vi "subPortInit.vi"(0 "Control unit ID":i32=1 min=1 max=10) -> (1 "Index":i32, 2 "InitOK":bool)   [LabVIEW 2018, in "DLOwis.lvclass"]
uses:
  DLOwis.lvclass
panel:
  in  "error in (no error)":errorcluster
  out "DLOwis.lvclass":refnum<class "DLOwis.lvclass">
  in  "DLOwis.lvclass":refnum<class "DLOwis.lvclass">
  in  "Timeout":i32 caption="Timeout, ms" min=0
  in  "Network port":u16=1200
  in  "ip4":u8 caption="IP address"
  in  "ip3":u8 caption="IP address"
  in  "ip2":u8 caption="IP address"
  in  "ip1":u8 caption="IP address"
  in  "logging on":bool
  in  "Delay":i32(slide) caption="Fast(0)<--->Slow(50)" min=0 max=50 scale=0.0..50.0
  in  "Baudrate":string(combo)="9600"
  in  "Cancel":bool
  in  "OK":bool
  in  "COM port":i32=-1 caption="COMx" min=-1 max=255
  out "Error":i32
  in  "Interface":bool
  # "Parameters of the interface"
  # "COMx=-1: find\nautomatically"
  # "IP=0.0.0.0: connect\n 1. local ip address \n and port 1200"
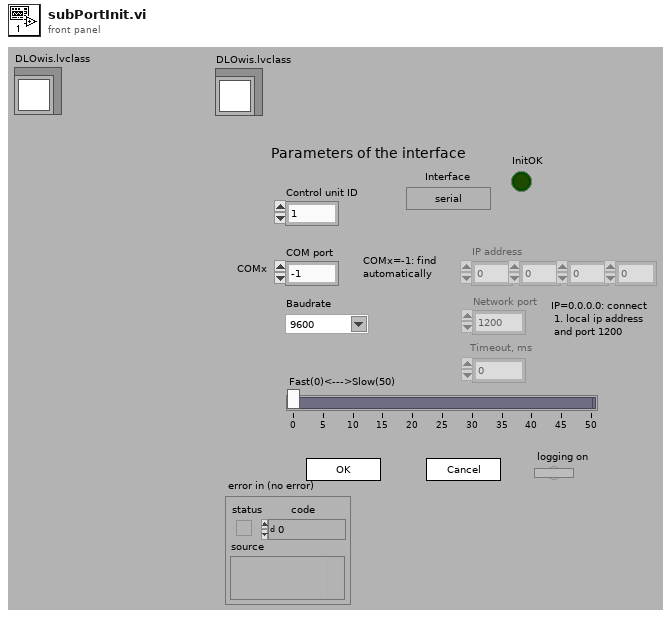
[diagram p1: front panel]
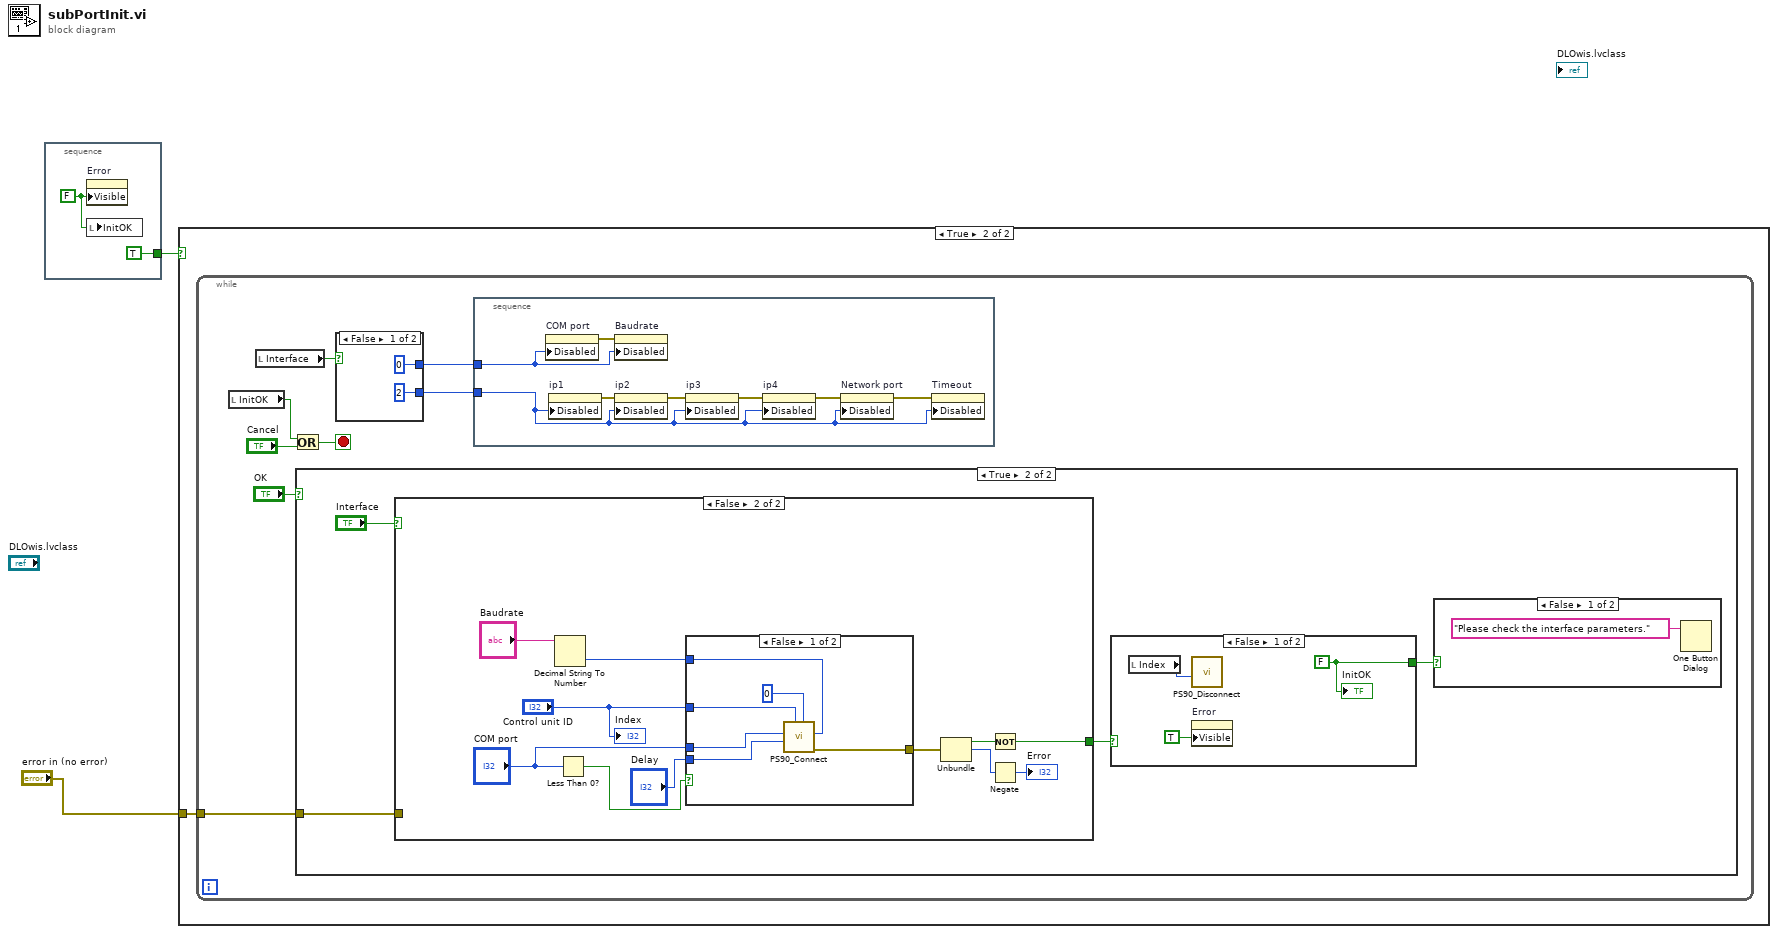
[diagram p0: block diagram]
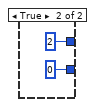
[diagram p3: hidden frame]
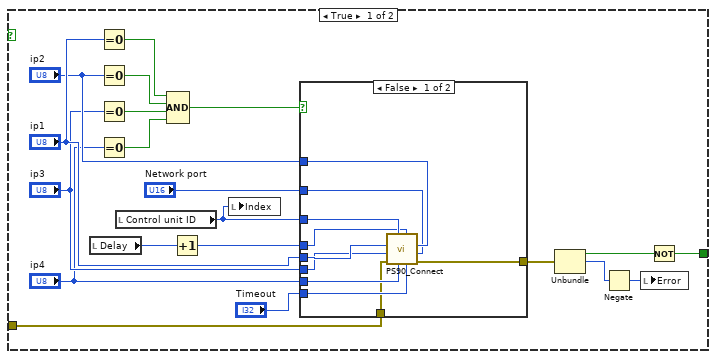
[diagram p5: hidden frame]
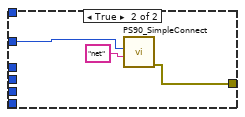
[diagram p6: hidden frame]
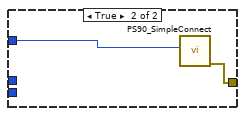
[diagram p7: hidden frame]
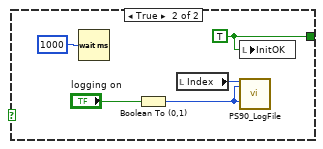
[diagram p8: hidden frame]
diagram:
  n1 = stacked-sequence {
    tunnel: [TRUE] -> w2
    frame #0 {
      w3 = FALSE ("Visible")
      n2 = property on="Error" class="DigNum (strict)"("Visible"=w3) -> ()  [unwired: 2 in, 2 out]
      n3 = local write "InitOK"(w3) -> ()
    }
  }
  n4 = case shown="True" w2 {
    tunnel: "error in (no error)" -> [_ w5]
    frame False {
    }
    frame True {
      n5 = while {
        tunnel: w5 -> [w6]
        stop <- w13 stop-if-true
        n6 = local read "InitOK"() -> (w10:bool)
        n7 = local read "Interface"() -> (w7:bool)
        n8 = Or(x=w10, y="Cancel") -> (x .or. y?=w13:bool)
        n9 = case shown="True" "OK" {
          tunnel: w6 -> [_ w26]
          frame False {
          }
          frame True {
            n10 = case shown="False" "Interface" {
              tunnel: [w45 w71] -> w28
              tunnel: w26 -> [w30 _]
              frame True {
                n11 = local read "Delay"() -> (w33:i32)
                n12 = Equal To 0?(x="ip1") -> (x = 0?=w42:bool)
                n13 = Equal To 0?(x="ip2") -> (x = 0?=w41:bool)
                n14 = Equal To 0?(x="ip3") -> (x = 0?=w39:bool)
                n15 = Equal To 0?(x="ip4") -> (x = 0?=w40:bool)
                n16 = local read "Control unit ID"() -> (w49:i32)
                n17 = Compound Arithmetic op=AND(w42, w41, w39, w40) -> (w43:bool)
                n18 = Increment(x=w33) -> (x+1=w32:i32)
                n19 = local write "Index"(w49) -> ()
                n20 = case shown="False" w43 {
                  tunnel: [w59 w62] -> w46
                  tunnel: w49 -> [w58 w61]
                  tunnel: "ip1" -> [w57 _]
                  tunnel: "ip2" -> [w56 _]
                  tunnel: "ip3" -> [w55 _]
                  tunnel: "ip4" -> [w54 _]
                  tunnel: "Network port" -> [w53 _]
                  tunnel: w32 -> [w52 _]
                  tunnel: "Timeout" -> [w51 _]
                  tunnel: w30 -> [w50 _]
                  frame False {
                    n21 = call "PS90_Connect.vi"("par5"=w53, "par2"=w56, "par6"=w51, "Interface"=w52, "par4"=w54, "Control unit ID"=w58, "error in (no error)"=w50, "par3"=w55, "par1"=w57) -> ("error out"=w59:errorcluster)  [unwired: 1 in, 1 out]
                  }
                  frame True {
                    n22 = call "PS90_SimpleConnect.vi"("Serial number"="net", "Control unit ID"=w61) -> ("error out"=w62:errorcluster)  [unwired: 8 in, 1 out]
                  }
                }
                n23 = Unbundle(w46) -> ("status"=w47:bool, "code"=w48:i32)  [unwired: 1 out]
                n24 = Negate(x=w48) -> (-x=w44:i32)
                n25 = local write "Error"(w44) -> ()
                n26 = Not(x=w47) -> (.not. x?=w45:bool)
              }
              frame False {
                n27 = Decimal String To Number(string="Baudrate") -> (number=w67:i32)  [unwired: 2 in, 1 out]
                n28 = Less Than 0?(x="COM port") -> (x < 0?=w64:bool)
                n29 = case shown="False" w64 {
                  tunnel: [w79 w81] -> w73
                  tunnel: "Control unit ID" -> [w77 w80]
                  tunnel: "COM port" -> [w76 _]
                  tunnel: w67 -> [w75 _]
                  tunnel: "Delay" -> [w74 _]
                  frame False {
                    n30 = call "PS90_Connect.vi"("par2"=w75, "Interface"=u32 0, "Control unit ID"=w77, "par3"=w74, "par1"=w76) -> ("error out"=w79:errorcluster)  [unwired: 5 in, 1 out]
                  }
                  frame True {
                    n31 = call "PS90_SimpleConnect.vi"("Control unit ID"=w80) -> ("error out"=w81:errorcluster)  [unwired: 9 in, 1 out]
                  }
                }
                n32 = Unbundle(w73) -> ("status"=w70:bool, "code"=w72:i32)  [unwired: 1 out]
                n33 = Not(x=w70) -> (.not. x?=w71:bool)
                n34 = Negate(x=w72) -> (-x=→"Error":i32)
                "Index" <- "Control unit ID"
              }
            }
            n35 = case shown="False" w28 {
              tunnel: [w82 w86] -> w29
              frame False {
                w82 = FALSE ("WriteOK")
                n36 = local read "Index"() -> (w83:i32)
                n37 = call "PS90_Disconnect.vi"("Control unit ID"=w83) -> ()  [unwired: 5 in, 2 out]
                n38 = property on="Error" class="DigNum (strict)"("Visible"=TRUE) -> ()  [unwired: 2 in, 2 out]
                "InitOK" <- w82
              }
              frame True {
                w86 = TRUE ("WriteOK")
                n39 = Wait (ms)(milliseconds to wait=u32 1000 ("Zu wartende ms")) -> ()  [unwired: 1 out]
                n40 = Boolean To (0,1)(Boolean="logging on") -> (0, 1=w85:i16)
                n41 = local read "Index"() -> (w88:i32)
                n42 = local write "InitOK"(w86) -> ()
                n43 = call "PS90_LogFile.vi"("Control unit ID"=w88, "nOpen"=w85, "Mode"=w85) -> ()  [unwired: 16 in, 1 out]
              }
            }
            n44 = case shown="False" w29 {
              frame False {
                n45 = One Button Dialog(message="Please check the interface parameters.") -> ()  [unwired: 1 in, 1 out]
              }
              frame True {
              }
            }
          }
        }
        n46 = case shown="False" w7 {
          tunnel: [0 2] -> w8
          tunnel: [2 0] -> w9
          frame False {
          }
          frame True {
          }
        }
        n47 = stacked-sequence {
          tunnel: w8 -> [w20]
          tunnel: w9 -> [w18]
          frame #0 {
            n48 = property on="COM port" class="DigNum (strict)"("Disabled"=w20) -> (error out=w21:errorcluster)  [unwired: 2 in, 1 out]
            n49 = property on="ip1" class="DigNum (strict)"("Disabled"=w18) -> (error out=w22:errorcluster)  [unwired: 2 in, 1 out]
            n50 = property on="Baudrate" class="CmbBox"(error in=w21, "Disabled"=w20) -> ()  [unwired: 1 in, 2 out]
            n51 = property on="ip2" class="DigNum (strict)"(error in=w22, "Disabled"=w18) -> (error out=w23:errorcluster)  [unwired: 1 in, 1 out]
            n52 = property on="ip3" class="DigNum (strict)"(error in=w23, "Disabled"=w18) -> (error out=w24:errorcluster)  [unwired: 1 in, 1 out]
            n53 = property on="ip4" class="DigNum (strict)"(error in=w24, "Disabled"=w18) -> (error out=w25:errorcluster)  [unwired: 1 in, 1 out]
            n54 = property on="Network port" class="DigNum (strict)"(error in=w25, "Disabled"=w18) -> (error out=w19:errorcluster)  [unwired: 1 in, 1 out]
            n55 = property on="Timeout" class="DigNum (strict)"(error in=w19, "Disabled"=w18) -> ()  [unwired: 1 in, 2 out]
          }
        }
      }
    }
  }
